vi "gHField.vi"() -> ()   [LabVIEW 2019]
panel:
  in  "Magnet System":enum16{"Resistive", "Hybrid"}(ring)
  in  "PS Setpoint":dbl format="%.2f"
  in  "PS Current":dbl format="%.2f"
  # "Field Controls"
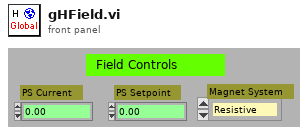
[diagram p1: front panel]
diagram:
